vi "ROI_mouse_checking.vi"(1 "input cluster":T2) -> (0 "output cluster":T1)   [LabVIEW 2010]
uses:
  <vilib>/Utility/inputDevices.llb/mouseAcquire.vi
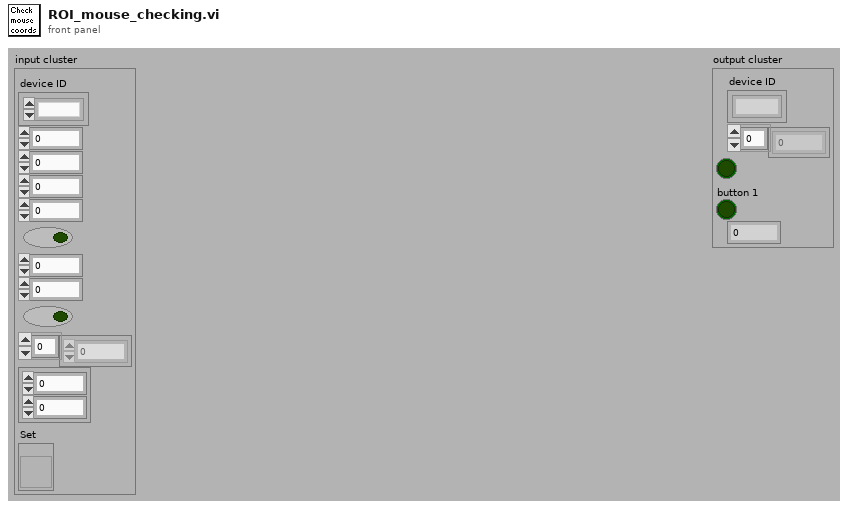
[diagram p1: front panel]
types:
  T1 = cluster{"device ID":refnum<k1>, dbl[], bool, "button 1":bool, i32}
  T2 = cluster{"device ID":refnum<k1>, i32, i32, u32, u32, bool, i32, i32, bool, dbl[], cluster{i32, i32}, "Set":refnum<vi>}
  T3 = cluster{"Horizontal":i32, "Vertical":i32, "Scrolling":i32}
  T4 = cluster{"button 1":bool, "button 2":bool, "button 3":bool, "button 4":bool}
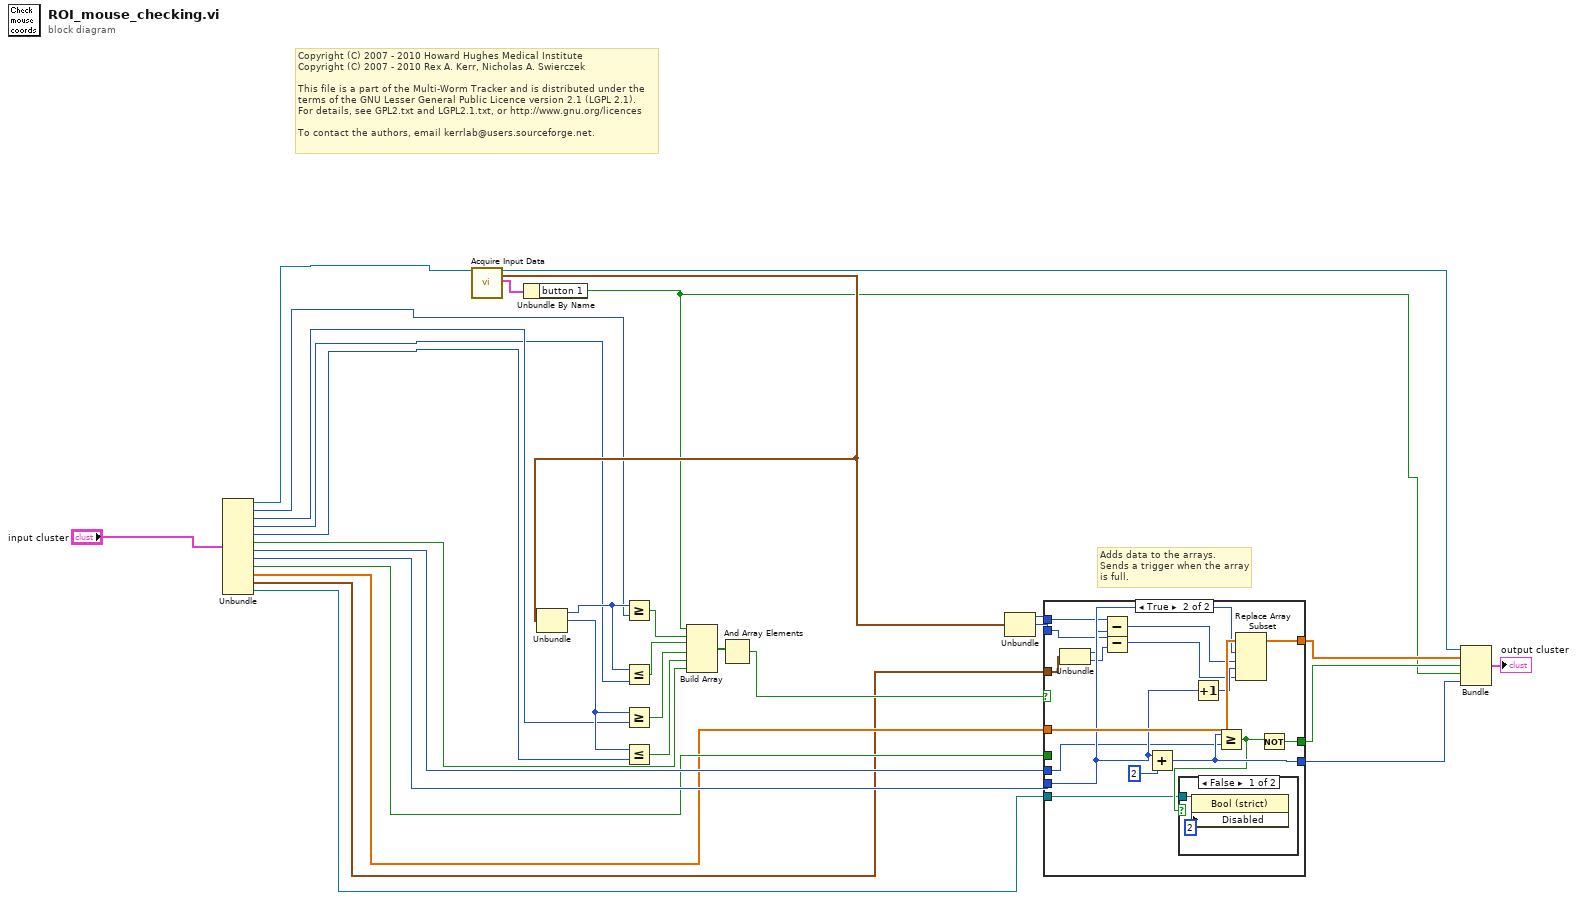
[diagram p0: block diagram]
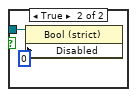
[diagram p3: hidden frame]
diagram:
  # "Copyright (C) 2007 - 2010 Howard Hughes Medical Institute\nCopyright (C) 2007 - 2010 Rex A. Kerr, Nicholas A. Swierczek\n \nThis file is a part of the Multi-Worm Tracker and is distributed under the\nterms of the GNU Lesser General Public Licence version 2.1 (LGPL 2.1).\nFor details, see GPL2.txt and LGPL2.1.txt, or http://www.gnu.org/licences\n \nTo contact the authors, email kerrlab@users.sourceforge.net."
  # "Adds data to the arrays.\nSends a trigger when the array\nis full."
  n1 = Unbundle("input cluster") -> ("device ID"=w20:refnum<k1>, w19:i32, w18:i32, w17:u32, w16:u32, w15:bool, w14:i32, w13:i32, w12:bool, w11:dbl[], w8:cluster{i32, i32}, "Set"=w4:refnum<vi>)
  n2 = call-poly <vilib>:"Acquire Input Data.vi"("device ID"=w20) -> ("device ID"=w6:refnum<k1>, "axis info"=w25:T3, "button info"=w7:T4)  [unwired: 15 in, 1 out]
  n3 = Unbundle By Name(w7) -> ("button 1"=w2:bool)
  n4 = Unbundle(w25) -> ("Horizontal"=w24:i32, "Vertical"=w23:i32)  [unwired: 1 out]
  n5 = Greater Or Equal?(x=w24, y=w19) -> (x >= y?=w31:bool)
  n6 = Less Or Equal?(x=w24, y=w17) -> (x <= y?=w30:bool)
  n7 = Greater Or Equal?(x=w23, y=w18) -> (x >= y?=w29:bool)
  n8 = Less Or Equal?(x=w23, y=w16) -> (x <= y?=w28:bool)
  n9 = Build Array(w2, w31, w30, w29, w28, w15) -> (w27:bool[])
  n10 = And Array Elements(Boolean array=w27) -> (logical AND=w26:bool)
  n11 = Unbundle(w25) -> ("Horizontal"=w22:i32, "Vertical"=w21:i32)  [unwired: 1 out]
  n12 = case shown="True" w26 {
    tunnel: w22 -> [_ w38]
    tunnel: w21 -> [_ w37]
    tunnel: w13 -> [w34 w48]
    tunnel: [w34 w46] -> w3
    tunnel: w11 -> [w33 w51]
    tunnel: [w33 w49] -> w9
    tunnel: w14 -> [_ w45]
    tunnel: [w32 w44] -> w10
    tunnel: w12 -> [w32 _]
    tunnel: w8 -> [_ w43]
    tunnel: w4 -> [_ w35]
    frame False {
    }
    frame True {
      n13 = Unbundle(w43) -> (w40:i32, w39:i32)
      n14 = Subtract(x=w38, y=w40) -> (x-y=w42:i32)
      n15 = Subtract(x=w37, y=w39) -> (x-y=w41:i32)
      n16 = Add(x=w48, y=2) -> (x+y=w46:i32)
      n17 = Increment(x=w48) -> (x+1=w50:i32)
      n18 = Greater Or Equal?(x=w46, y=w45) -> (x >= y?=w36:bool)
      n19 = case shown="False" w36 {
        tunnel: w35 -> [w52 w54]
        frame False {
          n20 = property on="Property Node" class="Bool (strict)"(reference=w52, "Disabled"=u8 2) -> ()  [unwired: 1 in, 2 out]
        }
        frame True {
          n21 = property on="Property Node" class="Bool (strict)"(reference=w54, "Disabled"=u8 0) -> ()  [unwired: 1 in, 2 out]
        }
      }
      n22 = Replace Array Subset(array=w51, new element #1=w42, index #1=w48, new element #2=w41, index #2=w50) -> (w49:dbl[])
      n23 = Not(x=w36) -> (.not. x?=w44:bool)
    }
  }
  n24 = Bundle("device ID"=w6, w9, w10, "button 1"=w2, w3) -> (→"output cluster":T1)  [unwired: 1 in]
